vi "Rotation Matrix to Quaternion.vi"(8 "error in (no error)":errorcluster, 11 "Rotation Matrix":T1) -> (0 "error out":errorcluster, 3 "Quaternion":T2)   [LabVIEW 2020, in "g_ar_toolkit.ar.lvlib"]
uses:
  g_ar_toolkit.ar.lvlib
  Quaternion.ctl
  <vilib>/Analysis/Matrix/Datatypes/RealMatrix.ctl
  g_ar_toolkit.common/g_ar_toolkit.common.lvlib
  <vilib>/Analysis/Matrix/NI_Matrix.lvlib
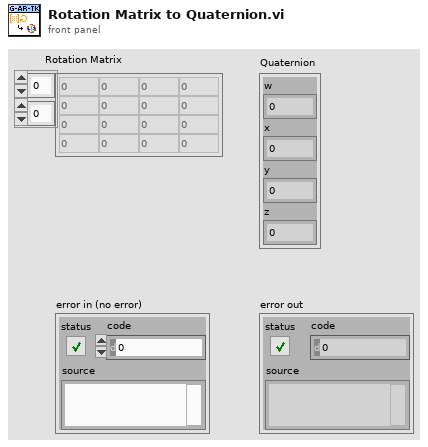
[diagram p1: front panel]
types:
  T1 = typedef "NI_Matrix.lvlib/RealMatrix.ctl" = dbl[][]
  T2 = typedef "g_ar_toolkit.ar.lvlib/Quaternion.ctl" = cluster{"w":dbl, "x":dbl, "y":dbl, "z":dbl}
  T3 = cluster{"Rotation Matrix[0]":dbl, "Rotation Matrix[1]":dbl, "Rotation Matrix[2]":dbl, "Rotation Matrix[3]":dbl, "Rotation Matrix[4]":dbl, "Rotation Matrix[5]":dbl, "Rotation Matrix[6]":dbl, "Rotation Matrix[7]":dbl, "Rotation Matrix[8]":dbl}
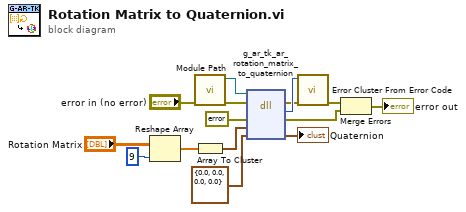
[diagram p0: block diagram]
diagram:
  n1 = Reshape Array("Rotation Matrix", 9 ("dimension size")) -> (w5:dbl[])
  n2 = call "Module Path.vi"("error in (no error)"="error in (no error)") -> ("error out"=w8:errorcluster, "Path"=w7:path)  [unwired: 9 in]
  n3 = Array To Cluster(array=w5) -> (cluster=w3:T3)
  n4 = dll-call lib="?" fn="g_ar_tk_ar_rotation_matrix_to_quaternion" ("g_ar_toolkit.*.*:g_ar_tk_image_copy")(path in=w7, error in=w8, "error_cluster"=errorcluster {"status"=FALSE, "code"=0, "source"=""} ("error constant"), "rmat"=w3, "quaternion"=T2 {"w"=0.0, "x"=0.0, "y"=0.0, "z"=0.0} ("Quaternion")) -> (error out=w10:errorcluster, "MgErr"=w11:i32, "error_cluster"=w14:errorcluster, "quaternion"=→"Quaternion":T2)  [unwired: 2 in, 1 out]
  n5 = call <vilib>:"Error Cluster From Error Code.vi"("error in (no error)"=w10, "error code (0)"=w11) -> ("error out"=w12:errorcluster)  [unwired: 7 in]
  n6 = Merge Errors(w12, w14) -> (→"error out":errorcluster)
